vi "writeAOchan_string_tt.vi"() -> (0 "AOchannel string":string, 1 "channelarray":bool[](array[boolean]))   [LabVIEW 2013]
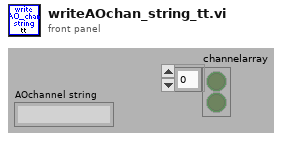
[diagram p1: front panel]
types:
  T1 = cluster{"Min Voltage (mV)":dbl, "Max voltage (mV)":dbl, "Duty cycle (%)":dbl, "Voltage freq. (Hz)":dbl, "# cycles":u32, "meastype":enum16{"sealtest hekcells", "sealtest neurons", "Manual", "from file"}, "sample rate":dbl, "Amplification (div10)":dbl, "sample mode":i32, "refreshbuffer":i32, "timeout":sgl, "patch":bool, "laserAO":bool, "shutter":bool, "488":bool, "532":bool, "640":bool}
  T2 = cluster{"CH1 AI":tag, "CH1 CI":tag, "CH2 AI":tag, "CH2 CI":tag, "AI X":tag, "AI Y":tag, "AO X-Y":tag, "CH1ST":bool, "CH2ST":bool, "Sigcase":i16, "StageS":i32, "StageL":i32, "data dir":path, "AI VC":tag, "AI CC":tag, "AO CWlaser":tag, "AO VtoP":tag, "shutter":tag, "488":tag, "532":tag, "640":tag}
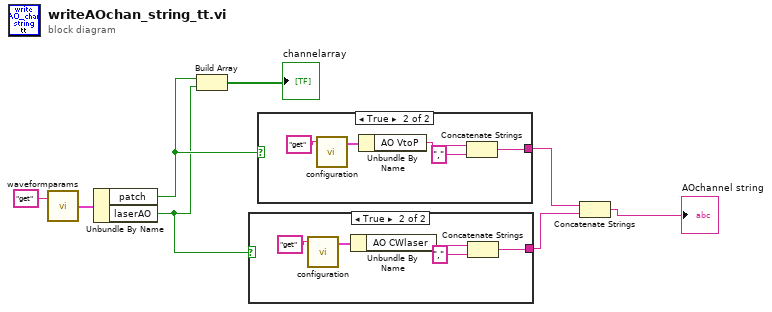
[diagram p0: block diagram]
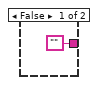
[diagram p2: hidden frame]
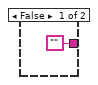
[diagram p3: hidden frame]
diagram:
  n1 = call "waveformparams.vi"("command"="get") -> ("Params out"=w5:T1)  [unwired: 1 in]
  n2 = Unbundle By Name(w5) -> ("patch"=w3:bool, "laserAO"=w2:bool)
  n3 = Build Array(w3, w2) -> (→"channelarray":bool[])
  n4 = case shown="True" w2 {
    tunnel: ["" w10] -> w7
    frame False {
    }
    frame True {
      n5 = call "configuration.vi"("command"="get") -> ("config out"=w13:T2)  [unwired: 2 in, 1 out]
      n6 = Unbundle By Name(w13) -> ("AO CWlaser"=w14:tag)
      n7 = Concatenate Strings(w14, ",") -> (w10:string)
    }
  }
  n8 = case shown="True" w3 {
    tunnel: ["" w16] -> w8
    frame False {
    }
    frame True {
      n9 = call "configuration.vi"("command"="get") -> ("config out"=w19:T2)  [unwired: 2 in, 1 out]
      n10 = Unbundle By Name(w19) -> ("AO VtoP"=w20:tag)
      n11 = Concatenate Strings(w20, ",") -> (w16:string)
    }
  }
  n12 = Concatenate Strings(w8, w7) -> (→"AOchannel string":string)
